vi "BindControlToMatlabValue.vi"(6 "Direction":T1, 8 "AllowVariantValues (f)":bool, 9 "Controls[]":refnum<vi>[](array[refnum]), 10 "Control":refnum<vi>, 11 "ExpID":string) -> ()   [LabVIEW 2017]
uses:
  Types/MatlabBindingDirectionEnum.ctl
  Types/ControlValueChangeEventBindingType.ctl
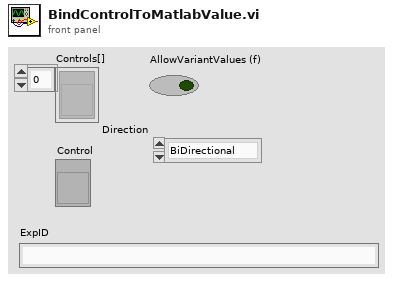
[diagram p1: front panel]
types:
  T1 = typedef "MatlabBindingDirectionEnum.ctl" = enum16{"BiDirectional", "FromMatlab", "ToMatlab"}
  T2 = typedef "ControlValueChangeEventBindingType.ctl" = cluster{"Control":refnum<vi>, "Event Register":refnum<event-registration>, "AllowVariantValues":bool, "Direction":T1, "Requires Update":bool, "Name":string}
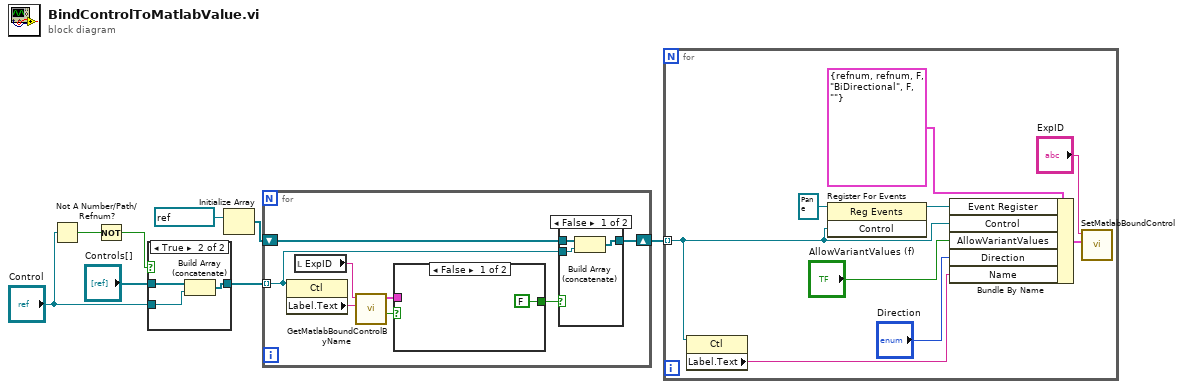
[diagram p0: block diagram]
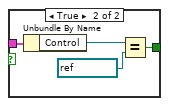
[diagram p2: hidden frame]
diagram:
  n1 = Not A Number/Path/Refnum?(number/path/refnum="Control") -> (NaN/Path/Refnum?=w8:bool)
  n2 = Not(x=w8) -> (.not. x?=w3:bool)
  n3 = case shown="True" w3 {
    tunnel: "Controls[]" -> [w9 w12]
    tunnel: "Control" -> [_ w11]
    tunnel: [w9 w10] -> w5
    frame False {
    }
    frame True {
      n4 = Build Array (concatenate)(w12, w11) -> (w10:refnum<vi>[])
    }
  }
  n5 = Initialize Array(refnum<vi> refnum ("Control")) -> (w1:refnum<vi>[])  [unwired: 1 in]
  n6 = for {
    tunnel: w5 -> [w13] mode=indexing
    shift-right: [w19] -> w4
    shift-left: w1 -> [w20]
    n7 = property class="Ctl"(reference=w13) -> ("Label.Text"=w14:string)  [unwired: 1 in, 2 out]
    n8 = local read "ExpID"() -> (w18:string)
    n9 = call "GetMatlabBoundControlByName.vi"("name"=w14, "ExperimentID"=w18) -> ("found"=w17:bool, "Control Binding"=w16:T2)  [unwired: 7 in, 1 out]
    n10 = case shown="False" w17 {
      tunnel: w16 -> [_ w25]
      tunnel: [FALSE w23] -> w15
      frame False {
      }
      frame True {
        n11 = Unbundle By Name(w25) -> ("Control"=w24:refnum<vi>)
        n12 = Equal?(x=w24, y=refnum<vi> refnum ("Control")) -> (x = y?=w23:bool)
      }
    }
    n13 = case shown="False" w15 {
      tunnel: w13 -> [w28 _]
      tunnel: w20 -> [w27 w29]
      tunnel: [w26 w29] -> w19
      frame False {
        n14 = Build Array (concatenate)(w27, w28) -> (w26:refnum<vi>[])
      }
      frame True {
      }
    }
  }
  n15 = for {
    tunnel: w4 -> [w33] mode=indexing
    n16 = property class="Ctl"(reference=w33) -> ("Label.Text"=w31:string)  [unwired: 1 in, 2 out]
    n17 = register-events(reference=refnum<event-registration> refnum ("event registration refnum"), w33) -> (reference out=w36:refnum<event-registration>)  [unwired: 1 in, 1 out]
    n18 = Bundle By Name(cluster=T2 {"Control"=refnum, "Event Register"=refnum, "AllowVariantValues"=FALSE, "Direction"=enum."BiDirectional", "Requires Update"=FALSE, "Name"=""}, "Event Register"=w36, "Control"=w33, "AllowVariantValues"="AllowVariantValues (f)", "Direction"="Direction", "Name"=w31) -> (w30:T2)
    n19 = call "SetMatlabBoundControl.vi"("Control Binding"=w30, "ExperimentID"="ExpID") -> ()  [unwired: 10 in]
  }
